vi "AddToQueue.vi"(0 "Cmd":string, 3 "ROS":T1, 4 "Type":enum16{"topic", "node", "ToFIFO", "ToWrite"}(ring)) -> (5 "ROS out":T1)   [LabVIEW 2014]
doc: "Adds ROS to the queue"
uses:
  <userlib>/ROS for LabVIEW Software.lnk/ROS/Code/SubVIs/_ROSControl.ctl
  <userlib>/ROS for LabVIEW Software.lnk/ROS/Code/SubVIs/_ROSDirection.ctl
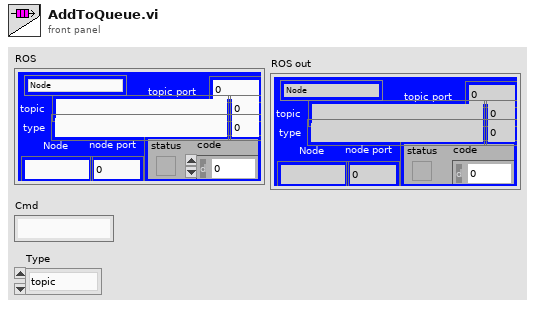
[diagram p1: front panel]
types:
  T1 = typedef "_ROSControl.ctl" = cluster{"topic port":u16, "Node":string, "topic":string, "type":string, "node port":u16, "error ":errorcluster, "Direction":T2, "Update (ms)":u16, "FIFO size":u16}
  T2 = typedef "_ROSDirection.ctl" = enum16{"Node", "Publisher", "Subscriber", "ServiceClient", "ServiceProvider"}
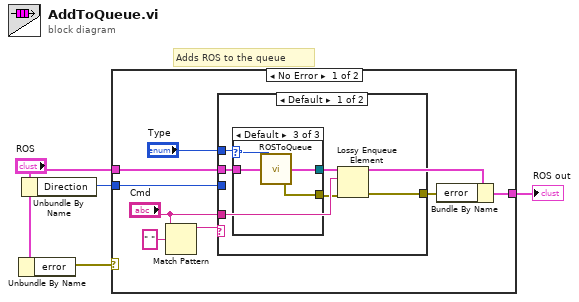
[diagram p0: block diagram]
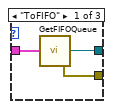
[diagram p2: hidden frame]
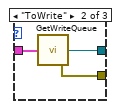
[diagram p3: hidden frame]
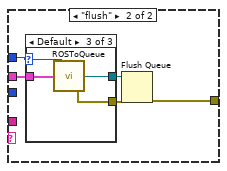
[diagram p4: hidden frame]
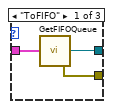
[diagram p5: hidden frame]
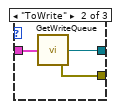
[diagram p6: hidden frame]
diagram:
  # "Adds ROS to the queue"
  n1 = Unbundle By Name("ROS") -> ("error"=w3:errorcluster)
  n2 = Unbundle By Name("ROS") -> ("Direction"=w1:T2)
  n3 = case shown="No Error" w3 {
    tunnel: "ROS" -> [w9 w44]
    tunnel: [w7 w44] -> w4
    tunnel: w1 -> [w5 _]
    frame No Error {
      n4 = Match Pattern(string="Cmd", regular expression=" ") -> (before substring=w10:string)  [unwired: 1 in, 3 out]
      n5 = case shown="Default" w10 {
        tunnel: "Cmd" -> [w18 _]
        tunnel: [w14 w33] -> w8
        tunnel: w9 -> [w17 w31]
        tunnel: "Type" -> [w15 w32]
        tunnel: w5 -> [_ _]
        frame Default {
          n6 = case shown="Default" w15 {
            selector: w15 -> [_ _ w26]
            tunnel: w17 -> [w21 w24 w28]
            tunnel: [w20 w22 w27] -> w16
            tunnel: [w19 w23 w25] -> w13
            frame "ToFIFO" {
              n7 = call <userlib>:"GetFIFOQueue.vi"("ROS"=w21) -> ("error out"=w19:errorcluster, "queue out"=w20:refnum<queue>)  [unwired: 3 in]
            }
            frame "ToWrite" {
              n8 = call <userlib>:"GetWriteQueue.vi"("ROS"=w24) -> ("error out"=w23:errorcluster, "queue out"=w22:refnum<queue>)  [unwired: 3 in]
            }
            frame Default {
              n9 = call <userlib>:"ROSToQueue.vi"("ROS"=w28, "Name"=w26) -> ("error out"=w25:errorcluster, "queue"=w27:refnum<queue>)  [unwired: 2 in]
            }
          }
          n10 = Lossy Enqueue Element(queue=w16, element=w18, error in (no error)=w13) -> (error out=w14:errorcluster)  [unwired: 3 out]
        }
        frame "flush" {
          n11 = case shown="Default" w32 {
            selector: w32 -> [_ _ w41]
            tunnel: w31 -> [w36 w39 w43]
            tunnel: [w35 w37 w42] -> w30
            tunnel: [w34 w38 w40] -> w29
            frame "ToFIFO" {
              n12 = call <userlib>:"GetFIFOQueue.vi"("ROS"=w36) -> ("error out"=w34:errorcluster, "queue out"=w35:refnum<queue>)  [unwired: 3 in]
            }
            frame "ToWrite" {
              n13 = call <userlib>:"GetWriteQueue.vi"("ROS"=w39) -> ("error out"=w38:errorcluster, "queue out"=w37:refnum<queue>)  [unwired: 3 in]
            }
            frame Default {
              n14 = call <userlib>:"ROSToQueue.vi"("ROS"=w43, "Name"=w41) -> ("error out"=w40:errorcluster, "queue"=w42:refnum<queue>)  [unwired: 2 in]
            }
          }
          n15 = Flush Queue(queue=w30, error in (no error)=w29) -> (error out=w33:errorcluster)  [unwired: 2 out]
        }
      }
      n16 = Bundle By Name(cluster=w9, "error"=w8) -> (w7:T1)
    }
    frame Error {
    }
  }
  "ROS out" <- w4
